vi "AudioGlobal.vi"() -> ()   [LabVIEW 2011]
panel:
  in  "TimeTraces":dbl[][](graph)=array2x72000[144000 elements]
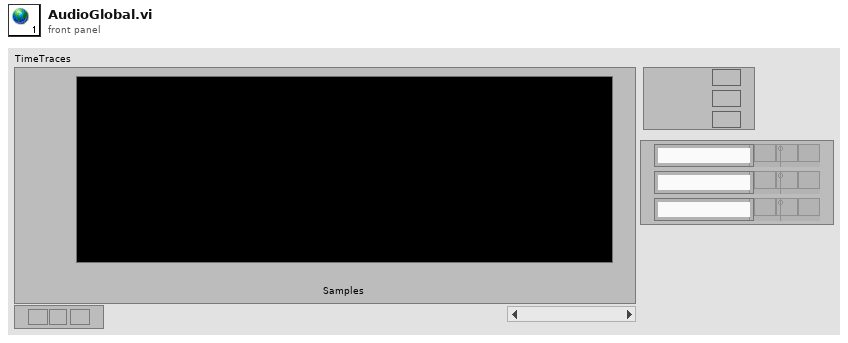
[diagram p1: front panel]
diagram:
